vi "Practica4.4_RegistrosForLoop.vi"() -> ()   [LabVIEW 2022 SP3]
panel:
  out "Datos":T1
  in  "CantEjecuciones":dbl
  out "Némero actual aleatorio":dbl(knob) scale=0.0..10.0
  out "Ultimo valor 11":dbl
  out "Ultimo valor 10":dbl
  out "Ultimo valor 9":dbl
  out "Ultimo valor 8":dbl
  out "Ultimo valor 7":dbl
  out "Ultimo valor 6":dbl
  out "Ultimo valor 5":dbl
  out "Ultimo valor 4":dbl
  out "Ultimo valor 3":dbl
  out "Ultimo valor 2":dbl
  out "Ejecuciones":dbl(knob) scale=0.0..50.0
  out "Ultimo valor 1":dbl
  out "Sí se encontró\nNo se encontró":bool
  in  "Valor selec":dbl
  # "Anahí Montserrat Vázquez Padilla \nPráctica 04: RegistrosForLoop\n07/02/2024"
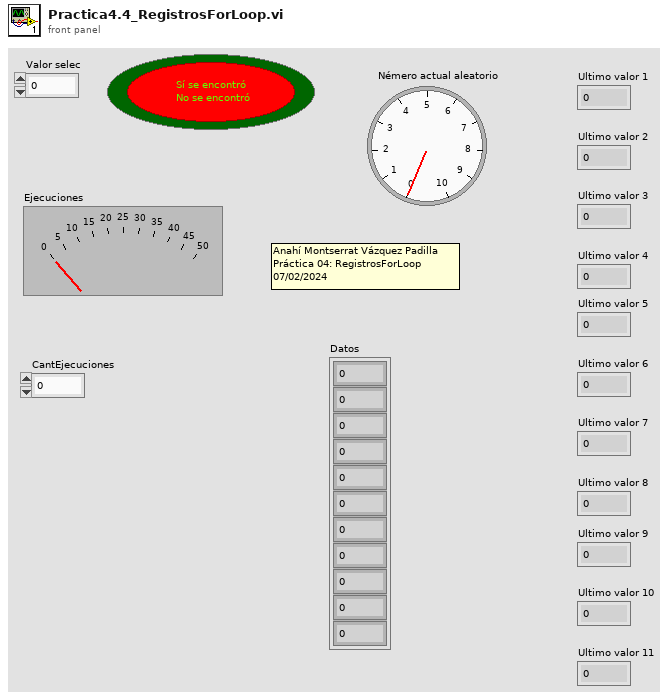
[diagram p1: front panel]
types:
  T1 = cluster{dbl, dbl, dbl, dbl, dbl, dbl, dbl, dbl, dbl, dbl, dbl}
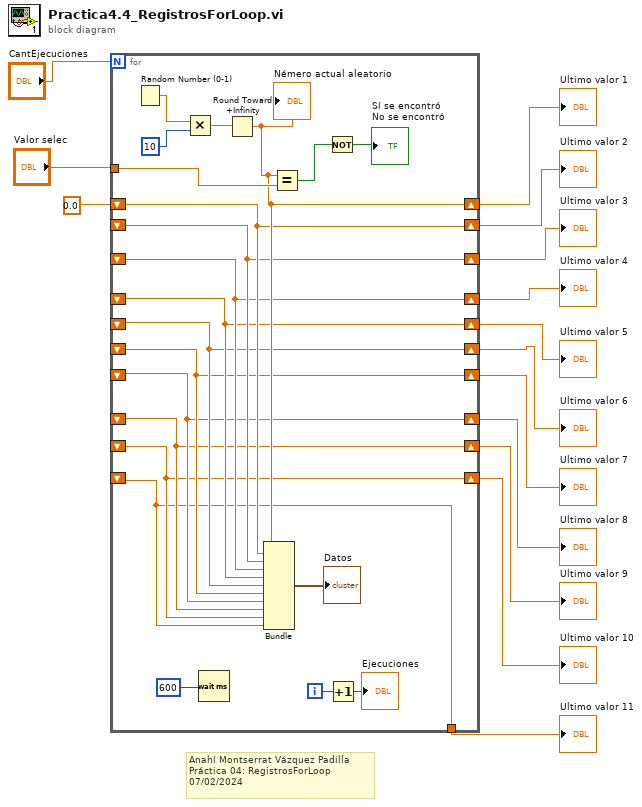
[diagram p0: block diagram]
diagram:
  # "Anahí Montserrat Vázquez Padilla \nPráctica 04: RegistrosForLoop\n07/02/2024"
  n1 = for {
    N: "CantEjecuciones" -> [_]
    tunnel: "Valor selec" -> [w32]
    shift-right: [w19] -> w6
    shift-left: _ -> [w18]
    shift-right: [w20] -> w7
    shift-left: _ -> [w19]
    shift-right: [w18] -> w5
    shift-left: _ -> [w17]
    shift-right: [w21] -> w8
    shift-left: _ -> [w20]
    shift-right: [w22] -> w9
    shift-left: _ -> [w21]
    shift-right: [w24] -> w11
    shift-left: _ -> [w23]
    shift-right: [w25] -> w12
    shift-left: _ -> [w24]
    shift-right: [w17] -> w4
    shift-left: _ -> [w16]
    shift-right: [w26] -> w13
    shift-left: 0.0 -> [w25]
    shift-right: [w23] -> w10
    shift-left: _ -> [w22]
    tunnel: [w16] -> w2
    i -> [w31]
    n2 = Random Number (0-1)() -> (number: 0 to 1=w34:dbl)
    n3 = Multiply(x=w34, y=10) -> (x*y=w33:dbl)
    n4 = Wait (ms)(milliseconds to wait=600) -> ()  [unwired: 1 out]
    n5 = Round Toward +Infinity(x=w33) -> (ceil(x): smallest int >= x=w26:dbl)
    "Némero actual aleatorio" <- w26
    n6 = Bundle(w26, w25, w24, w23, w22, w21, w20, w19, w18, w17, w16) -> (→"Datos":T1)  [unwired: 1 in]
    n7 = Equal?(x=w26, y=w32) -> (x = y?=w28:bool)
    n8 = Not(x=w28) -> (.not. x?=→"Sí se encontró\nNo se encontró":bool)
    n9 = Increment(x=w31) -> (x+1=→"Ejecuciones":i32)
  }
  "Ultimo valor 1" <- w13
  "Ultimo valor 2" <- w12
  "Ultimo valor 3" <- w11
  "Ultimo valor 4" <- w10
  "Ultimo valor 5" <- w9
  "Ultimo valor 6" <- w8
  "Ultimo valor 7" <- w7
  "Ultimo valor 8" <- w6
  "Ultimo valor 9" <- w5
  "Ultimo valor 10" <- w4
  "Ultimo valor 11" <- w2
